vi "DAQ@AnalogOutWaveForm__Parameter.vi"(1 "ParamterIn":string) -> (0 "ParamterOut":string)   [LabVIEW 2019]
panel:
  in  "WaveFrom":string(combo)
  in  "DAQName":string(combo)
  in  "Confirm":bool
  # "DAQ@AnalogOut $DAQ,$Voltage\nDAQ@AnalogOutWaveForm $DAQ,$WavefromName"
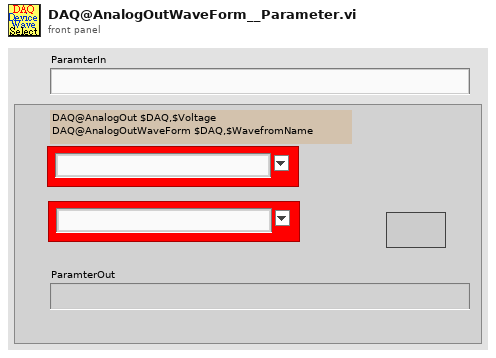
[diagram p1: front panel]
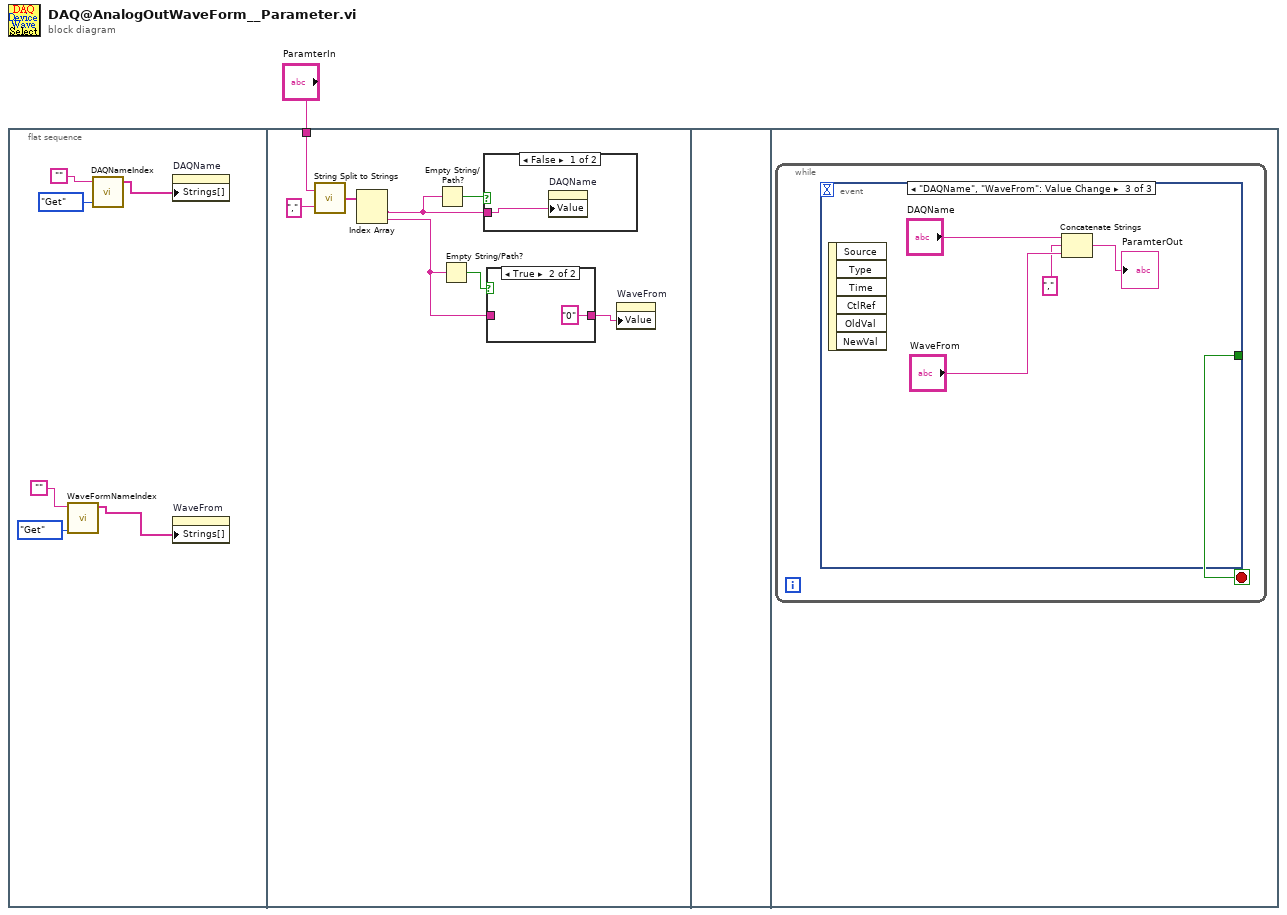
[diagram p0: block diagram]
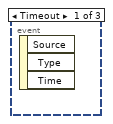
[diagram p4: hidden frame]
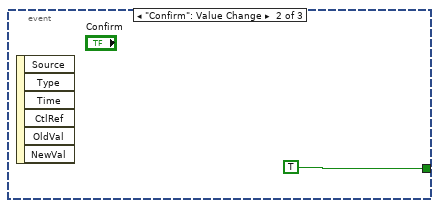
[diagram p5: hidden frame]
diagram:
  n1 = flat-sequence {
    tunnel: "ParamterIn" -> [w12]
    frame #0 {
      n2 = call "WaveFormNameIndex.vi"("OP"=enum16{"Get", "Update", "Init", "GetSPS"}."Get", "WaveFormName"="") -> ("WaveFormNameList"=w2:string[])  [unwired: 6 in, 3 out]
      n3 = call "DAQNameIndex.vi"("OP"=enum16{"Get", "Update", "Init"}."Get", "DAQName"="") -> ("DAQList"=w5:string[])  [unwired: 1 in, 2 out]
      n4 = property on="DAQName" class="CmbBox"("Strings[]"=w5) -> ()  [unwired: 2 in, 2 out]
      n5 = property on="WaveFrom" class="CmbBox"("Strings[]"=w2) -> ()  [unwired: 2 in, 2 out]
    }
    frame #1 {
      n6 = call "String Split to Strings.vi"("search string/char (-)"=",", "String"=w12) -> ("Array"=w14:string[])
      n7 = Index Array(array=w14) -> (element #1=w11:string, element #2=w8:string)  [unwired: 2 in]
      n8 = Empty String/Path?(string/path=w11) -> (empty?=w15:bool)
      n9 = Empty String/Path?(string/path=w8) -> (empty?=w10:bool)
      n10 = case shown="False" w15 {
        tunnel: w11 -> [w18 _]
        frame False {
          n11 = property on="DAQName" class="CmbBox"("Value"=w18) -> ()  [unwired: 2 in, 2 out]
        }
        frame True {
        }
      }
      n12 = case shown="True" w10 {
        tunnel: [w16 "0" ("ParamterIn")] -> w9
        tunnel: w8 -> [w16 _]
        frame False {
        }
        frame True {
        }
      }
      n13 = property on="WaveFrom" class="CmbBox"("Value"=w9) -> ()  [unwired: 2 in, 2 out]
    }
    frame #2 {
    }
    frame #3 {
      n14 = while {
        stop <- w19 stop-if-true
        n15 = event shown="[2] \"DAQName\", \"WaveFrom\": Value Change" {
          selector: _ -> [_ _ _]
          dyn-events: _ -> [_ _ _]
          timeout: _ -> [_ _ _]
          tunnel: [_ TRUE _] -> w19
          event Timeout {
            n16 = event-data() -> ()  [unwired: 1 in, 3 out]
          }
          event "Confirm": Value Change {
            n17 = event-data() -> ()  [unwired: 1 in, 6 out]
          }
          event "DAQName", "WaveFrom": Value Change {
            n18 = event-data() -> ()  [unwired: 1 in, 6 out]
            n19 = Concatenate Strings("DAQName", ",", "WaveFrom") -> (→"ParamterOut":string)
          }
        }
      }
    }
  }
